vi "test - value with Special Char.vi"(8 "error in (no error)":errorcluster, 11 "TestCase in":refnum<class "csm-ini-variable-addon.lvclass">) -> (0 "error out":errorcluster, 3 "TestCase out":refnum<class "csm-ini-variable-addon.lvclass">)   [LabVIEW 2017, in "csm-ini-variable-addon.lvclass"]
uses:
  csm-ini-variable-addon.lvclass
  bf93d063-bc2e-4fed-99a8-9cb4ff00e4c6.vi
  <userlib>/_NEVSTOP/Communicable State Machine(CSM)/addons/API-String-Arugments-Support/_Support/Convert API String Arguments to Data(variant).vi
  <vilib>/addons/_JKI Toolkits/VI Tester/TestCase.llb/TestCase.lvclass
  INI-Static-Variable-Support/INI-Static-Variable-Support.lvlib
  <userlib>/_NEVSTOP/Communicable State Machine(CSM)/addons/API-String-Arugments-Support/API String Arguments Support.lvlib
  C:/Program Files (x86)/National Instruments/LabVIEW 2017/vi.lib/addons/_JKI Toolkits/VI Tester/TestCase.llb/TestCase.lvclass
panel:
  out "String out":string
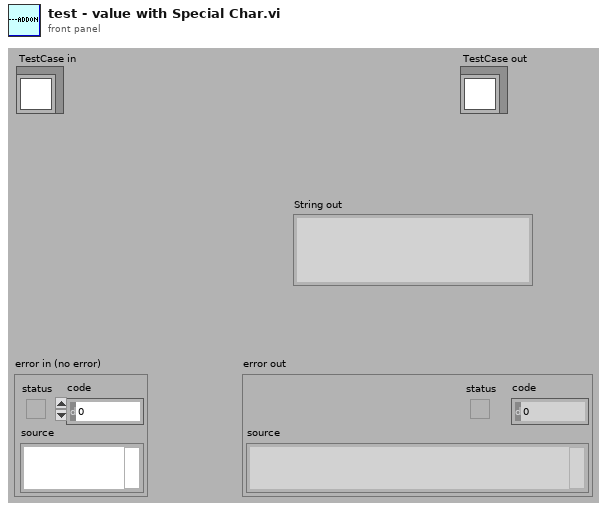
[diagram p1: front panel]
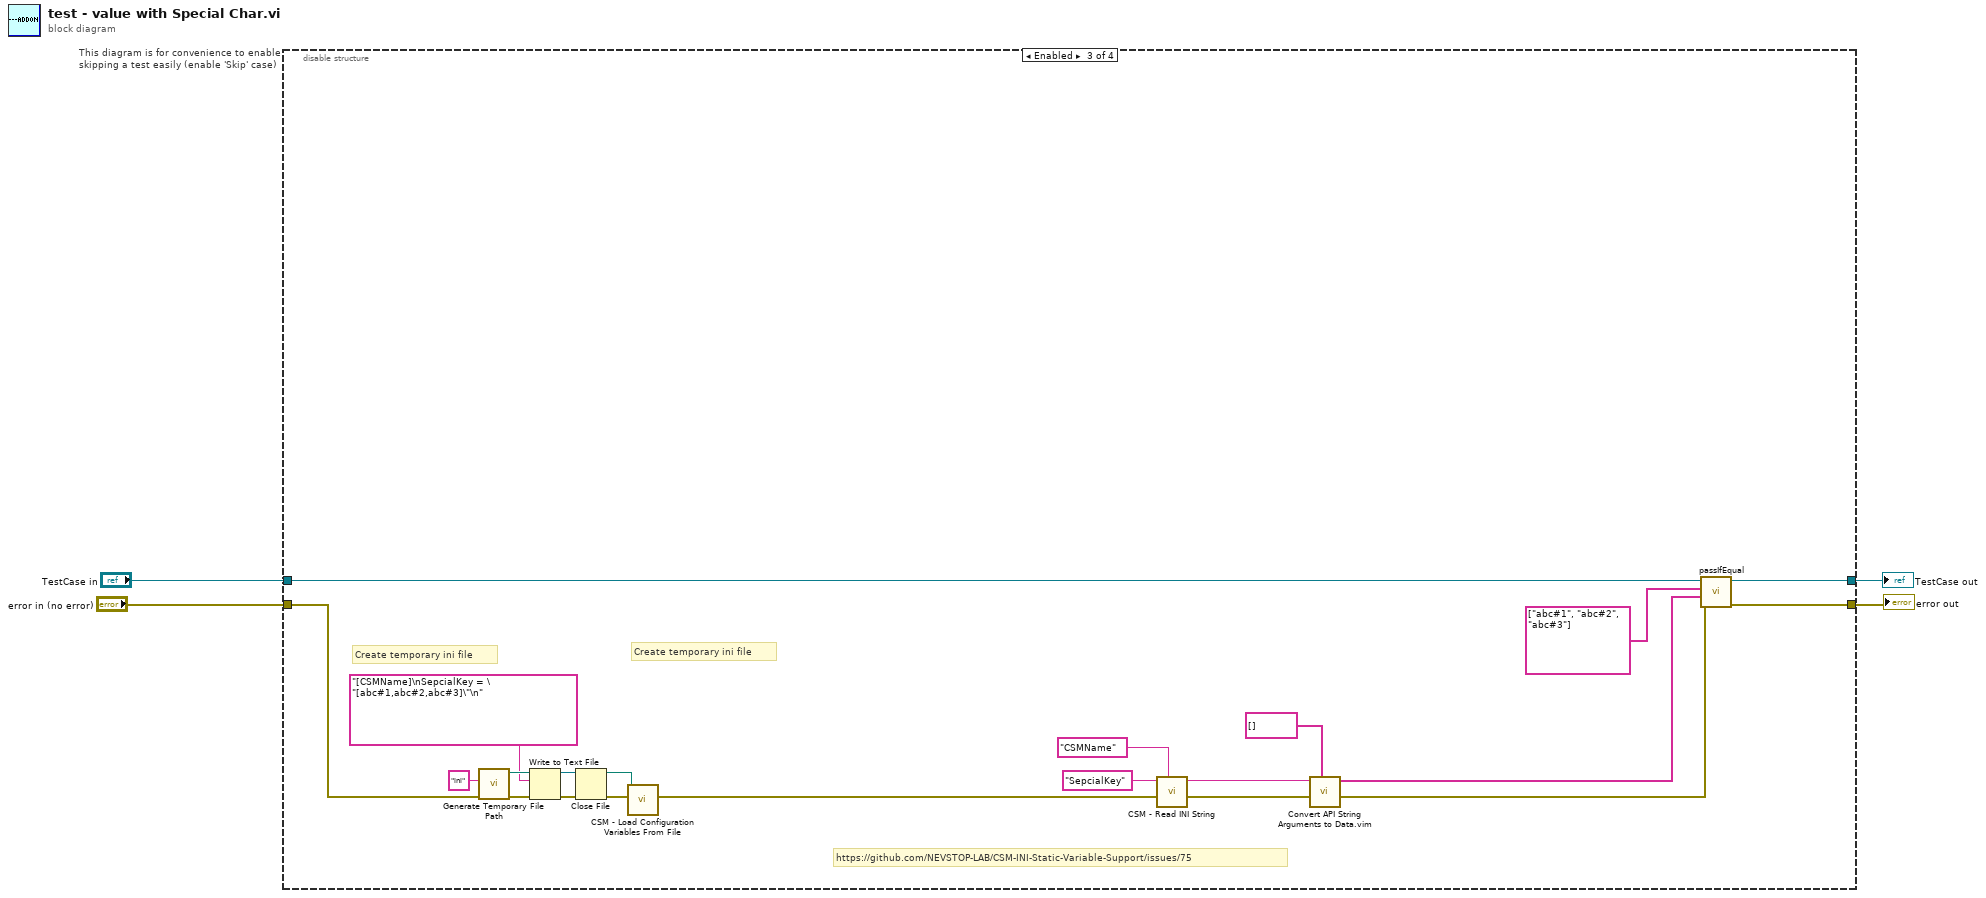
[diagram p0: block diagram]
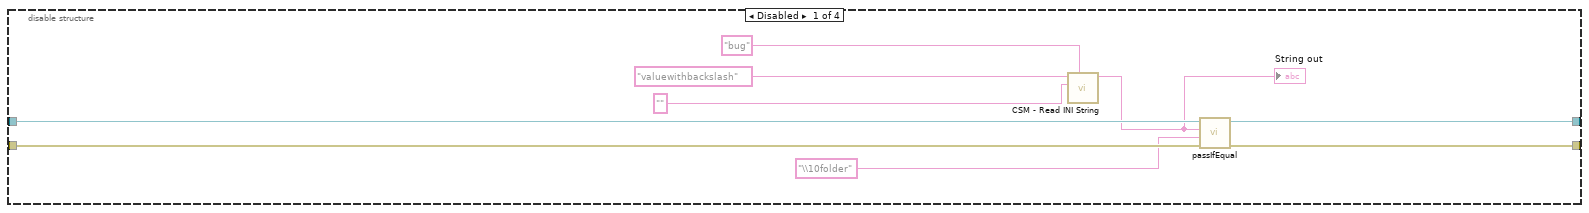
[diagram p2: hidden frame]
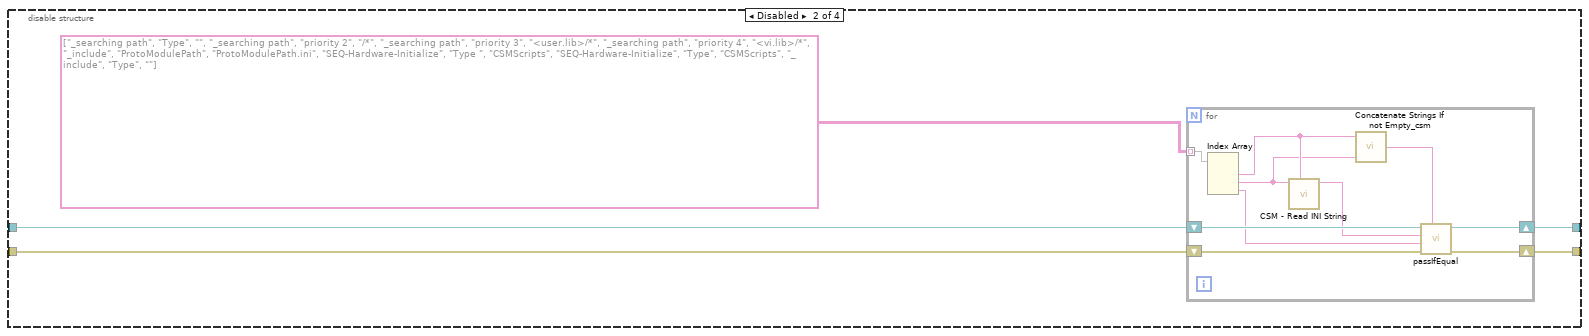
[diagram p3: hidden frame]
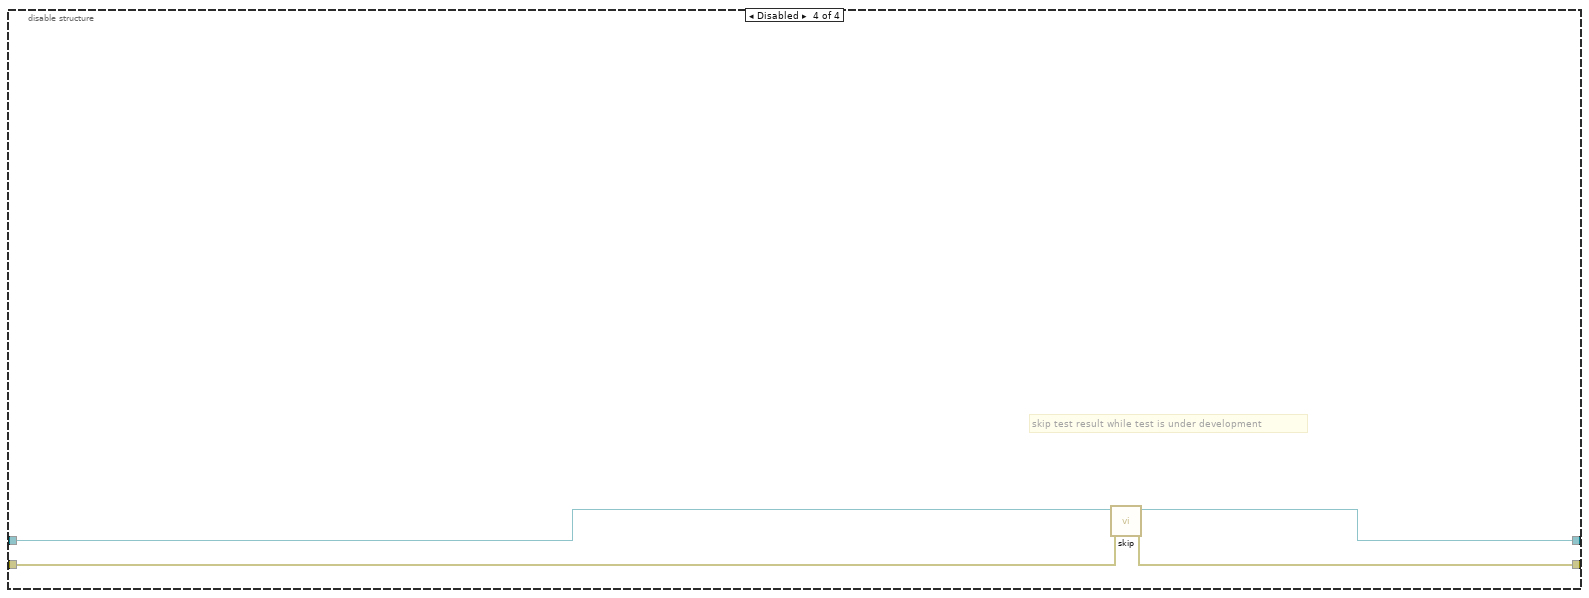
[diagram p4: hidden frame]
diagram:
  n1 = disable-structure "This diagram is for convenience to enable skipping a test easily (enable 'Skip' case)" shown="Enabled" {
    disable-tunnel: "TestCase in" -> [w10 w15 w39 w53]
    disable-tunnel: [w13 w18 w38 w51] -> w1
    disable-tunnel: [w12 w17 w29 w52] -> w3
    disable-tunnel: "error in (no error)" -> [w11 w16 w41 w50]
    frame Disabled {
      n2 = call "CSM - Read INI String.vi"("Section Name(\"\" as Default)"="bug" ("Section Name(\"\" as Default)"), ">> Default Value >>"="" ("String in"), "String in"="valuewithbackslash") -> ("String out"=w6:string)  [unwired: 4 in, 2 out]
      "String out" <- w6
      n3 = call-dynamic "passIfEqual.vi"("error in (no error)"=w11, "y"="\\10folder" ("String in"), "x"=w6, "TestCase in"=w10) -> ("error out"=w12:errorcluster, "TestCase out"=w13:refnum<class "csm-ini-variable-addon.lvclass">)  [unwired: 6 in]
    }
    frame Disabled {
      n4 = for {
        shift-right: [w27] -> w17
        shift-left: w16 -> [w26]
        shift-right: [w28] -> w18
        shift-left: w15 -> [w25]
        tunnel: string[][] [["_searching path", "Type", ""], ["_searching path", "priority 2", "/*"], ["_searching path", "priority 3", "<user.lib>/*"], ["_searching path", "priority 4", "<vi.lib>/*"], ["_include", "ProtoModulePath", "ProtoModulePath.ini"], ["SEQ-Hardware-Initialize", "Type ", "CSMScripts"], ["SEQ-Hardware-Initialize", "Type", "CSMScripts"], ["_include", "Type", ""]] -> [w23] mode=indexing
        n5 = Index Array(array=w23) -> (element #1=w20:string, element #2=w19:string, element #3=w22:string)  [unwired: 3 in]
        n6 = call "CSM - Read INI String.vi"("Section Name(\"\" as Default)"=w20, "String in"=w19) -> ("String out"=w24:string)  [unwired: 5 in, 2 out]
        n7 = call <userlib>:"Concatenate Strings If not Empty_csm.vi"("String"=w19, "prefix"=w20) -> ("result"=w21:string)  [unwired: 3 in]
        n8 = call-dynamic "passIfEqual.vi"("custom report message (\"\")"=w21, "error in (no error)"=w26, "y"=w22, "x"=w24, "TestCase in"=w25) -> ("error out"=w27:errorcluster, "TestCase out"=w28:refnum<class "csm-ini-variable-addon.lvclass">)  [unwired: 5 in]
      }
    }
    frame Enabled {
      # "https://github.com/NEVSTOP-LAB/CSM-INI-Static-Variable-Support/issues/75"
      # "Create temporary ini file"
      # "Create temporary ini file"
      n9 = call <vilib>:"Generate Temporary File Path.vi"("error in (no error)"=w41, "Temporary File Extension (tmp)"="ini") -> ("error out"=w49:errorcluster, "Unique Temporary File Path"=w46:path)  [unwired: 8 in]
      n10 = Write to Text File(file (use dialog)=w46, text="[CSMName]\nSepcialKey = \"[abc#1,abc#2,abc#3]\"\n", error in=w49) -> (refnum out=w45:refnum<file>, error out=w47:errorcluster)  [unwired: 1 in, 1 out]
      n11 = Close File(refnum=w45, error in=w47) -> (path=w42:path, error out=w44:errorcluster)
      n12 = call "CSM - Load Configuration Variables From File.vi"("error in (no error)"=w44, "Path"=w42) -> ("error out"=w40:errorcluster)  [unwired: 7 in]
      n13 = call "CSM - Read INI String.vi"("Section Name(\"\" as Default)"="CSMName" ("Section Name(\"\" as Default)"), "error in (no error)"=w40, "String in"="SepcialKey") -> ("error out"=w37:errorcluster, "String out"=w34:string)  [unwired: 4 in, 1 out]
      n14 = call "Convert API String Arguments to Data.vim"("Type"=string[] [] ("String in"), "error in (no error)"=w37, "String"=w34) -> ("error"=w30:errorcluster, "Data"=w31:string[])  [unwired: 5 in]
      n15 = call-dynamic "passIfEqual.vi"("error in (no error)"=w30, "y"=w31, "x"=string[] ["abc#1", "abc#2", "abc#3"] ("String in"), "TestCase in"=w39) -> ("error out"=w29:errorcluster, "TestCase out"=w38:refnum<class "csm-ini-variable-addon.lvclass">)  [unwired: 6 in]
    }
    frame Disabled {
      # "skip test result while test is under development"
      n16 = call <vilib>:"skip.vi"("error in (no error)"=w50, "TestCase in"=w53) -> ("error out"=w52:errorcluster, "TestCase out"=w51:refnum<class "csm-ini-variable-addon.lvclass">)  [unwired: 8 in]
    }
  }
  "error out" <- w3
  "TestCase out" <- w1
